vi "process_error_location.vi"(11 "Error in":refnum<class "Error.lvclass">) -> (3 "error_source_object":string)   [LabVIEW 2023, in "Error Handling Interface.lvlib" / "Error.lvclass"]
doc: "From the object definition, identifies the error location.\nTo be used by the Error class to decode the source actor/object"
uses:
  Error.lvclass
  Error.lvclass/Error.ctl
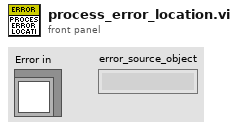
[diagram p1: front panel]
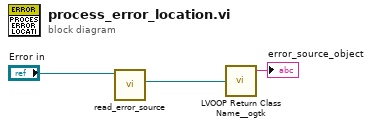
[diagram p0: block diagram]
diagram:
  n1 = call "read_error_source.vi"("Error in"="Error in") -> ("error_source"=w1:refnum<class>)  [unwired: 10 in]
  n2 = call <userlib>:"LVOOP Return Class Name__ogtk.vi"("Object"=w1) -> ("Class Base Name"=→"error_source_object":string)  [unwired: 2 out]
